vi "loadingpattern.vi"() -> ()   [LabVIEW 2022 SP3]
uses:
  <vilib>/DAQmx/write.llb/DAQmx Write (Digital 1D Bool 1Chan 1Samp).vi
  <vilib>/DAQmx/create/channels.llb/DAQmx Create Channel (DO-Digital Output).vi
  <vilib>/DAQmx/miscellaneous.llb/DAQmx Fill In Error Info.vi
panel:
  in  "Light Pattern (leftmost light=top button, rightmost light=bottom button)":bool[](array[boolean])=[TRUE, FALSE, FALSE, FALSE, FALSE, FALSE, FALSE, FALSE]
  in  "Backwards Mode (Forwards moves the light left to right)":bool
  in  "Start on LED(1= leftmost LED, 8= Rightmost LED)":dbl=1.0
  in  "Between X Leds (Greater than 1)":dbl=8.0
  out "Iteration":dbl
  out "error out":errorcluster
  in  "stop":bool
  in  "LED Flashing Rate (flashes per second)\nInput a Number from 1 to 500":i32=5
  # "Loading Screen Pattern"
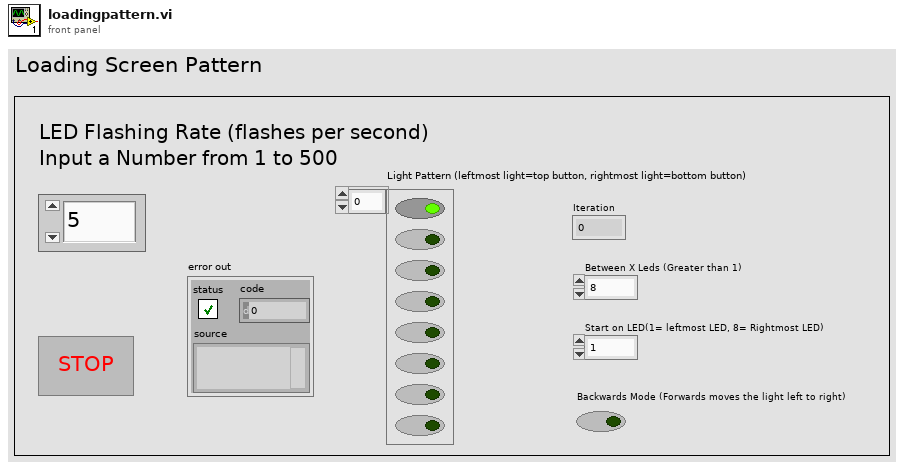
[diagram p1: front panel]
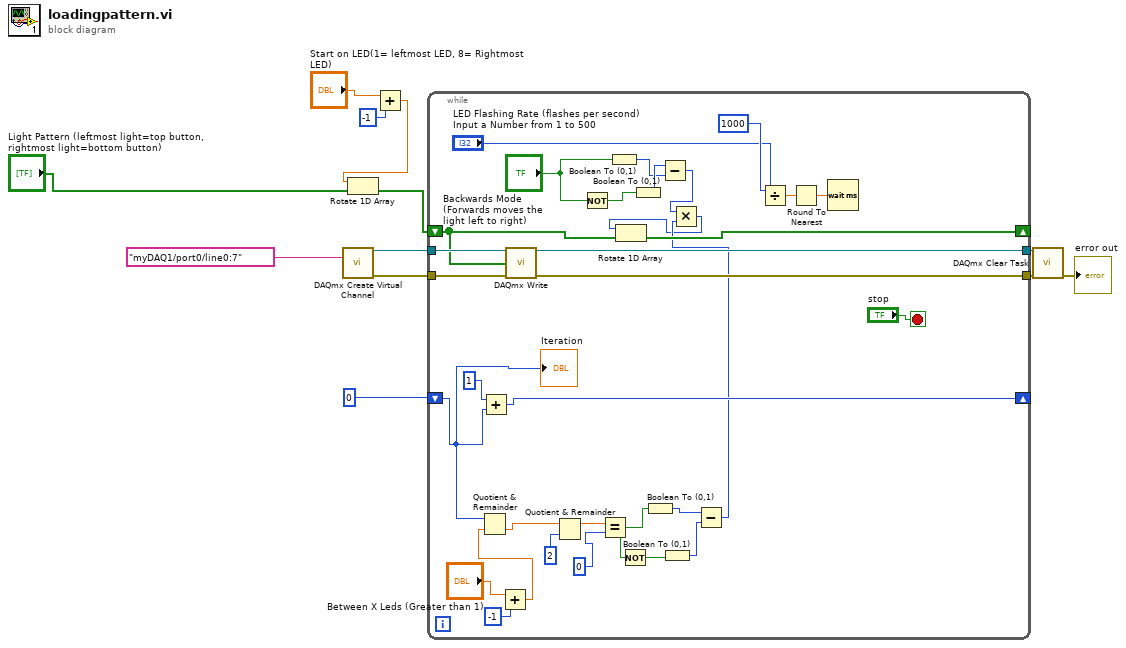
[diagram p0: block diagram]
diagram:
  n1 = call-poly <vilib>:"DAQmx Create Virtual Channel.vi"("lines"=tag "myDAQ1/port0/line0:7") -> ("task out"=w11:refnum<k21>, "error out"=w10:errorcluster)  [unwired: 13 in]
  n2 = Add(x="Start on LED(1= leftmost LED, 8= Rightmost LED)", y=-1) -> (x+y=w2:dbl)
  n3 = Rotate 1D Array(1:"Light Pattern (leftmost light=top button, rightmost light=bottom button)", 2:w2) -> (0:w5:bool[])
  n4 = while {
    shift-right: [w35] -> _
    shift-left: w5 -> [w34]
    tunnel: w11 -> [w39]
    tunnel: w10 -> [w38]
    tunnel: [w37] -> w9
    tunnel: [w36] -> w8
    shift-right: [w32] -> _
    shift-left: 0 -> [w23]
    stop <- "stop" stop-if-true
    n5 = Add(x=1, y=w23) -> (x+y=w32:i32)
    n6 = Add(x="Between X Leds (Greater than 1)", y=-1) -> (x+y=w20:dbl)
    n7 = Quotient & Remainder(x=w23, y=w20) -> (floor(x/y)=w30:dbl)  [unwired: 1 out]
    n8 = call-poly <vilib>:"DAQmx Write.vi"("task/channels in"=w39, "data"=w34, "error in"=w38) -> ("task out"=w37:refnum<k21>, "error out"=w36:errorcluster)  [unwired: 10 in, 1 out]
    n9 = Quotient & Remainder(x=w30, y=2) -> (x-y*floor(x/y)=w28:dbl)  [unwired: 1 out]
    n10 = Not(x="Backwards Mode (Forwards moves the light left to right)") -> (.not. x?=w19:bool)
    n11 = Equal?(x=w28, y=0) -> (x = y?=w24:bool)
    n12 = Boolean To (0,1)(Boolean="Backwards Mode (Forwards moves the light left to right)") -> (0, 1=w16:i16)
    n13 = Not(x=w24) -> (.not. x?=w27:bool)
    n14 = Boolean To (0,1)(Boolean=w19) -> (0, 1=w17:i16)
    n15 = Boolean To (0,1)(Boolean=w24) -> (0, 1=w25:i16)
    n16 = Subtract(x=w17, y=w16) -> (x-y=w15:i16)
    n17 = Boolean To (0,1)(Boolean=w27) -> (0, 1=w26:i16)
    n18 = Subtract(x=w25, y=w26) -> (x-y=w14:i16)
    n19 = Multiply(x=w15, y=w14) -> (x*y=w13:i16)
    n20 = Rotate 1D Array(1:w34, 2:w13) -> (0:w35:bool[])
    n21 = Divide(x=1000, y="LED Flashing Rate (flashes per second)\nInput a Number from 1 to 500") -> (x/y=w41:dbl)
    n22 = Round To Nearest(number=w41) -> (nearest integer value=w40:dbl)
    n23 = Wait (ms)(milliseconds to wait=w40) -> ()  [unwired: 1 out]
    "Iteration" <- w23
  }
  n24 = call <vilib>:"DAQmx Clear Task.vi"("task in"=w9, "error in"=w8) -> ("error out"=→"error out":errorcluster)  [unwired: 13 in]
